vi "Plot axis key focus set.vi"(8 "error in (no error)":errorcluster, 10 "target axis":T1, 11 "Refs":T2) -> (0 "error out":errorcluster)   [LabVIEW 2021, in "RocketPlot.lvlib"]
uses:
  RocketPlot.lvlib
  TypeDefs/Plot UI references.ctl
  Classes/RocketPlotHandle/RocketPlotHandle.lvclass
  <userlib>/bjustice/TipStripOOPanel/Classes/TipPanelHandle/TipPanelHandle.lvclass
  TypeDefs/Plot top row.ctl
  TypeDefs/Plot axis.ctl
  Plot scale refnum to LUT name.vi
  FormatStringTime.vi
  Plot AxisFocus position.vi
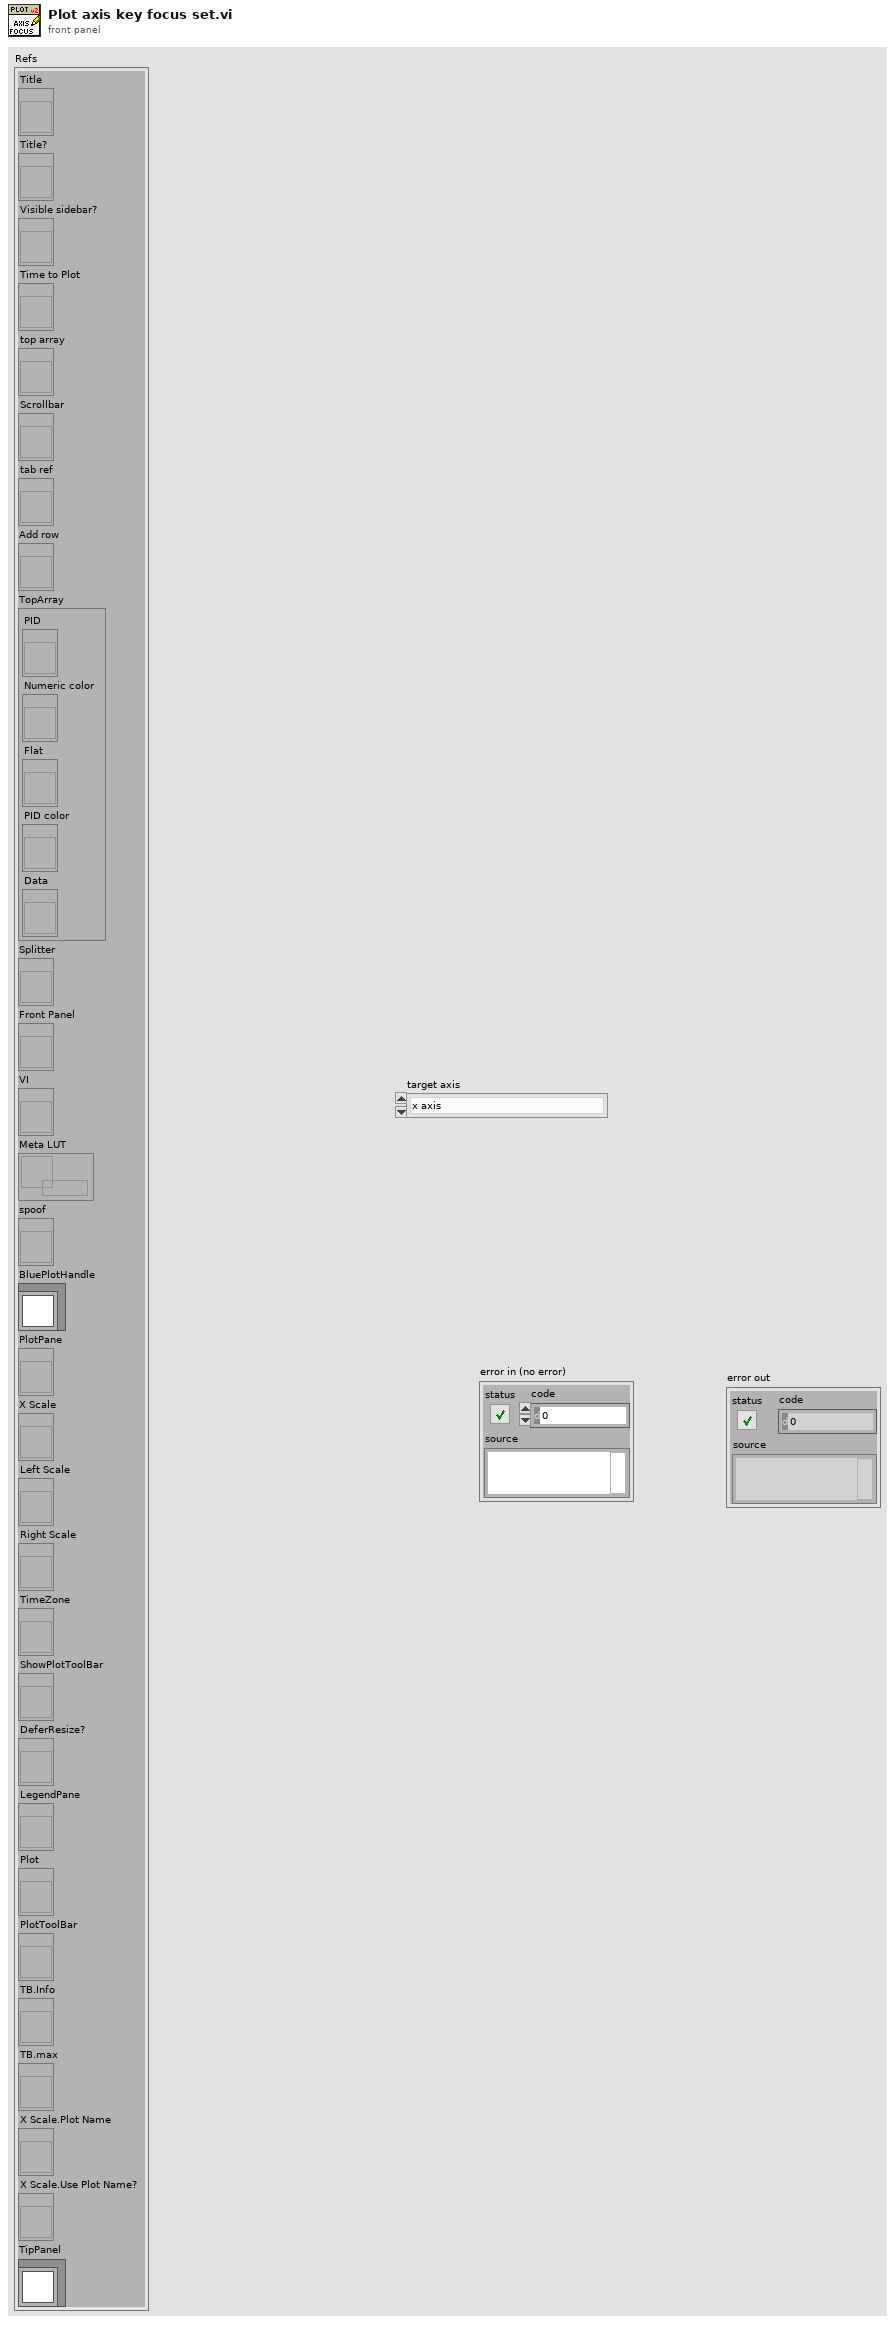
[diagram p1: front panel]
types:
  T1 = typedef "RocketPlot.lvlib/Plot axis.ctl" = enum16{"x axis", "left axis", "right axis"}
  T2 = typedef "RocketPlot.lvlib/Plot UI references.ctl" = cluster{"Title":refnum<vi>, "Title?":refnum<vi>, "Visible sidebar?":refnum<vi>, "Time to Plot":refnum<vi>, "top array":refnum<vi>, "Scrollbar":refnum<vi>, "tab ref":refnum<vi>, "Add row":refnum<vi>, "TopArray":cluster{"PID":refnum<vi>, "Numeric color":refnum<vi>, "Flat":refnum<vi>, "PID color":refnum<vi>, "Data":refnum<vi>}, "Splitter":refnum<vi>, "Front Panel":refnum<vi>, "VI":refnum<vi>, "Meta LUT":refnum<data-value>, "spoof":refnum<vi>, "BluePlotHandle":refnum<class "RocketPlotHandle.lvclass">, "PlotPane":refnum<vi>, "X Scale":refnum<vi>, "Left Scale":refnum<vi>, "Right Scale":refnum<vi>, "TimeZone":refnum<vi>, "ShowPlotToolBar":refnum<vi>, "DeferResize?":refnum<vi>, "LegendPane":refnum<vi>, "Plot":refnum<vi>, "PlotToolBar":refnum<vi>, "TB.Info":refnum<vi>, "TB.max":refnum<vi>, "X Scale.Plot Name":refnum<vi>, "X Scale.Use Plot Name?":refnum<vi>, "TipPanel":refnum<class "TipPanelHandle.lvclass">}
  T3 = typedef "TimeZone.ctl" = enum16{"UTC", "Local"}
  T4 = typedef "RocketPlot.lvlib/Plot scale meta JSON.ctl" = cluster{"Type":T1, "Grid Colors:Major Color":u32, "Grid Colors:Minor Color":u32, "Style":u8, "Tick Colors:Tick Color":u32, "Tick Colors:Minor Tick Color":u32, "Format String":string, "State":T5, "AxisFocus":refnum<vi>}
  T5 = typedef "RocketPlot.lvlib/Plot scale meta state.ctl" = cluster{"Visible":bool, "Focus":bool, "Multi-Y":bool}
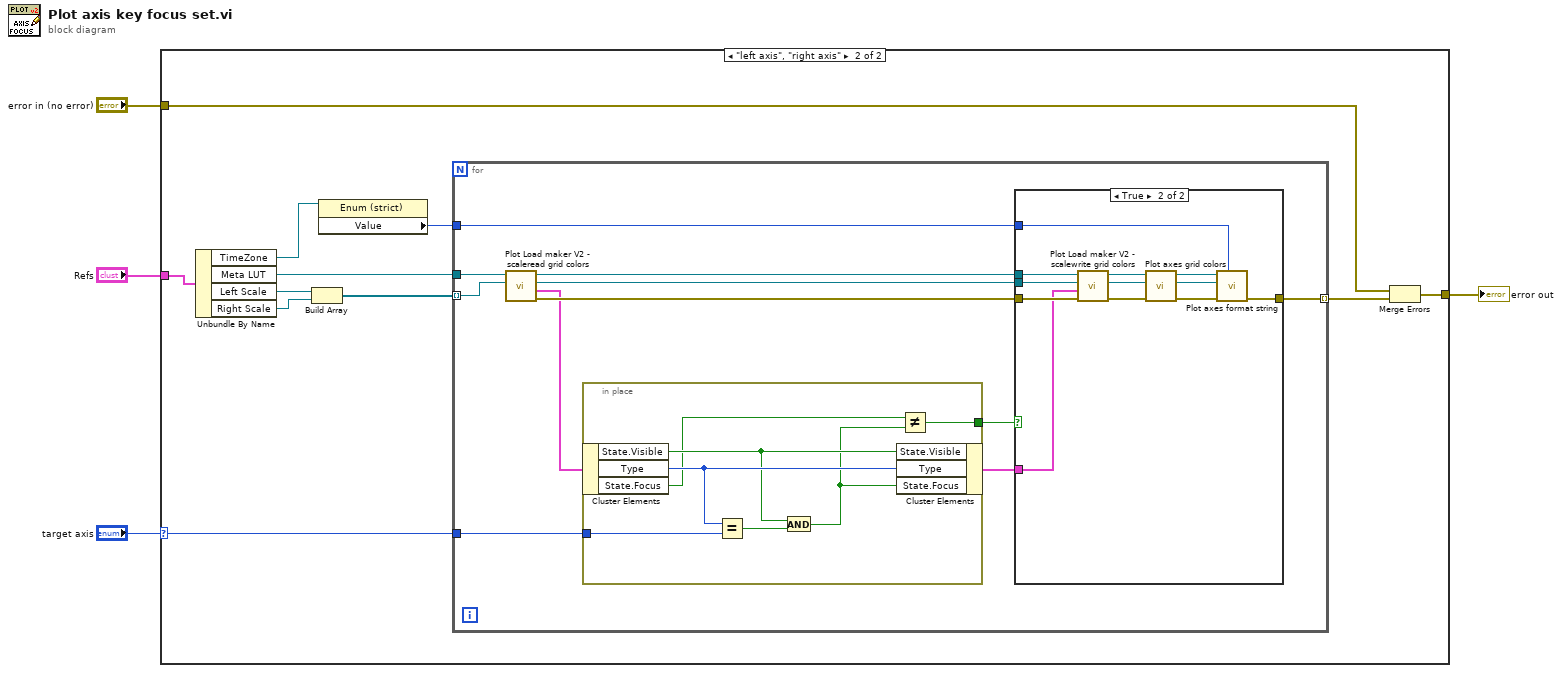
[diagram p0: block diagram]
diagram:
  n1 = case shown="\"left axis\", \"right axis\"" "target axis" {
    selector: "target axis" -> [_ w14]
    tunnel: "Refs" -> [_ w16]
    tunnel: "error in (no error)" -> [w5 w9]
    tunnel: [w5 w8] -> w1
    frame "x axis" {
    }
    frame "left axis", "right axis" {
      n2 = Unbundle By Name(w16) -> ("TimeZone"=w6:refnum<vi>, "Meta LUT"=w15:refnum<data-value>, "Left Scale"=w13:refnum<vi>, "Right Scale"=w12:refnum<vi>)
      n3 = Build Array(w13, w12) -> (w11:refnum<vi>[])
      n4 = property class="Enum (strict)"(reference=w6) -> ("Value"=w7:T3)  [unwired: 1 in, 2 out]
      n5 = for {
        tunnel: w15 -> [w27]
        tunnel: w14 -> [w25]
        tunnel: w11 -> [w22] mode=indexing
        tunnel: [w21] -> w10 mode=indexing
        tunnel: w7 -> [w20]
        n6 = call "Plot Load maker V2 - scaleread grid colors.vi"("Scale reference"=w22, "Meta LUT"=w27) -> ("error out"=w24:errorcluster, "Scale LUT meta"=w18:T4, "Scale reference"=w23:refnum<vi>, "Meta LUT"=w26:refnum<data-value>)  [unwired: 6 in]
        n7 = in-place {
          in-place-border: w25 -> [w47]
          in-place-border: [w41] -> w17
          n8 = in-place-cluster #1(w18) -> ("State.Visible"=w44:bool, "Type"=w45:T1, "State.Focus"=w43:bool)
          n9 = Equal?(x=w45, y=w47) -> (x = y?=w46:bool)
          n10 = And(x=w44, y=w46) -> (x .and. y?=w42:bool)
          n11 = in-place-cluster #1("State.Visible"=w44, "Type"=w45, "State.Focus"=w42) -> (w19:T4)
          n12 = Not Equal?(x=w43, y=w42) -> (x != y?=w41:bool)
        }
        n13 = case shown="True" w17 {
          tunnel: w26 -> [_ w40]
          tunnel: w24 -> [w28 w39]
          tunnel: w23 -> [_ w38]
          tunnel: [w28 w31] -> w21
          tunnel: w20 -> [_ w29]
          tunnel: w19 -> [_ w30]
          frame False {
          }
          frame True {
            n14 = call "Plot Load maker V2 - scalewrite grid colors.vi"("error in (no error)"=w39, "Meta"=w30, "Scale reference"=w38, "Meta LUT"=w40) -> ("error out"=w36:errorcluster, "Scale reference"=w37:refnum<vi>, "Meta LUT"=w35:refnum<data-value>)  [unwired: 5 in]
            n15 = call "Plot axes grid colors.vi"("error in (no error)"=w36, "Scale reference"=w37, "Meta LUT"=w35) -> ("error out"=w34:errorcluster, "Scale reference"=w32:refnum<vi>, "Meta LUT"=w33:refnum<data-value>)  [unwired: 6 in]
            n16 = call "Plot axes format string.vi"("TimeZone"=w29, "error in (no error)"=w34, "Scale reference"=w32, "Meta LUT"=w33) -> ("error out"=w31:errorcluster)  [unwired: 6 in, 1 out]
          }
        }
      }
      n17 = Merge Errors(w9, w10) -> (w8:errorcluster)
    }
  }
  "error out" <- w1
